vi "Read Gains Message.vi"(8 "error in (no error)":errorcluster, 11 "PID Gains Set Message in":refnum<class "PID Gains Set Message.lvclass">) -> (0 "error out":errorcluster, 2 "Gains":T1 {"D (Td)" format="%#_9f"; "I (Ti)" format="%#_9f"; "P (Kc)" format="%#.9f"}, 3 "PID Gains Set Message out":refnum<class "PID Gains Set Message.lvclass">)   [LabVIEW 2015, in "RDS Child Messages.lvlib" / "PID Gains Set Message.lvclass"]
uses:
  PID Gains Set Message.lvclass
  PID Gains Control.ctl
  PID Gains Set Message.lvclass/PID Gains Set Message.ctl
  RDS Child Messages.lvlib
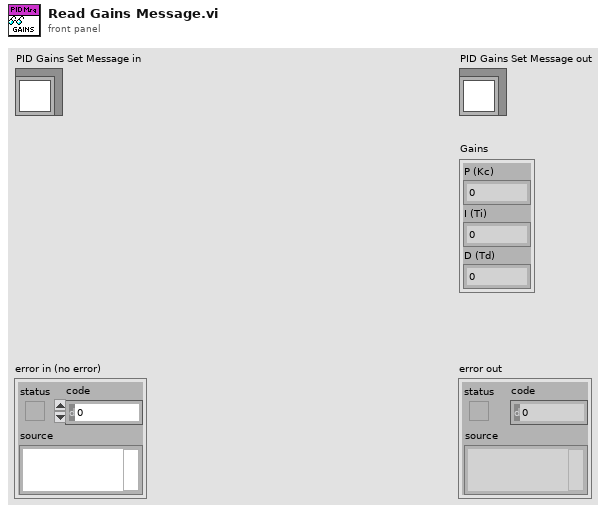
[diagram p1: front panel]
types:
  T1 = typedef "RDS Child Messages.lvlib/PID Gains Control.ctl" = cluster{"P (Kc)":sgl, "I (Ti)":sgl, "D (Td)":sgl}
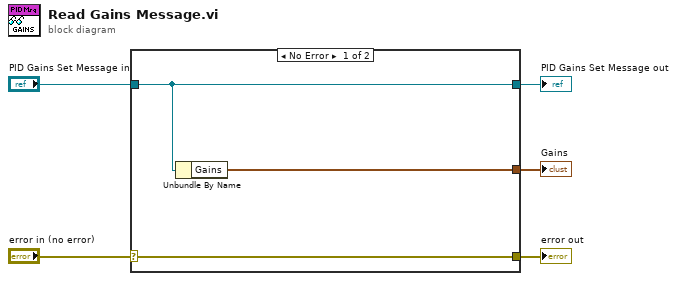
[diagram p0: block diagram]
diagram:
  n1 = case shown="No Error" "error in (no error)" {
    selector: "error in (no error)" -> [w8 w9]
    tunnel: [w8 w9] -> w4
    tunnel: [w7 w10] -> w2
    tunnel: "PID Gains Set Message in" -> [w7 w10]
    tunnel: [w6 _] -> w1
    frame No Error {
      n2 = Unbundle By Name(w7) -> ("Gains"=w6:T1)
    }
    frame Error {
    }
  }
  "error out" <- w4
  "PID Gains Set Message out" <- w2
  "Gains" <- w1
